vi "smartmeshIP serial mux check connection.vi"(8 "error in":errorcluster, 11 "serial mux adress":T1={"serial_mux IP"="127.0.0.1", "rserial_mux port"=9900}) -> (0 "error out":errorcluster, 3 "last error out connection":errorcluster)   [LabVIEW 2017]
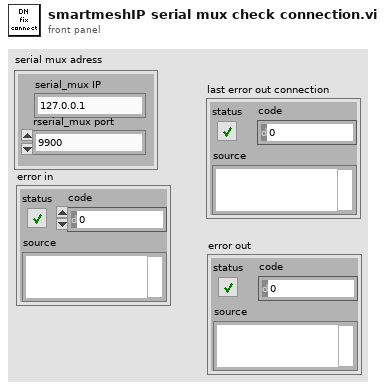
[diagram p1: front panel]
types:
  T1 = cluster{"serial_mux IP":string, "rserial_mux port":u16}
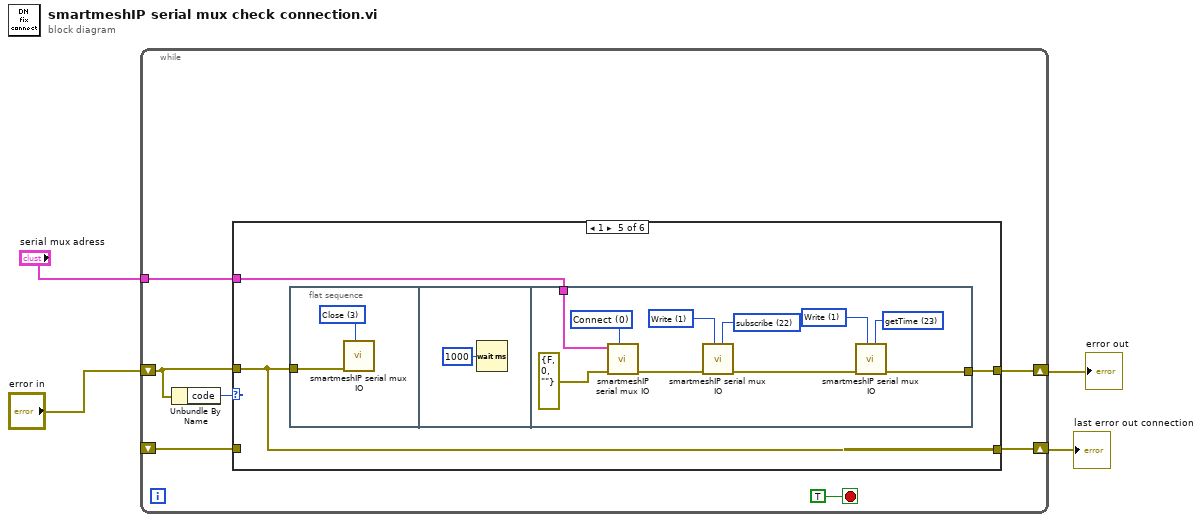
[diagram p0: block diagram]
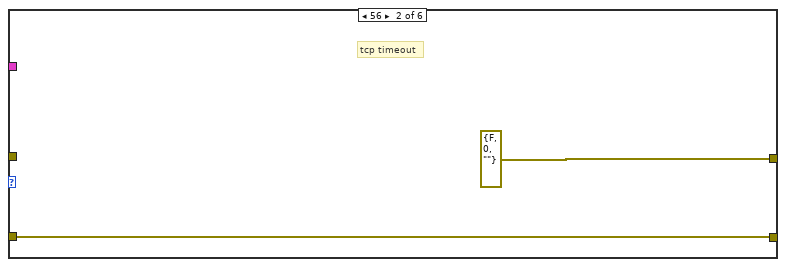
[diagram p3: hidden frame]
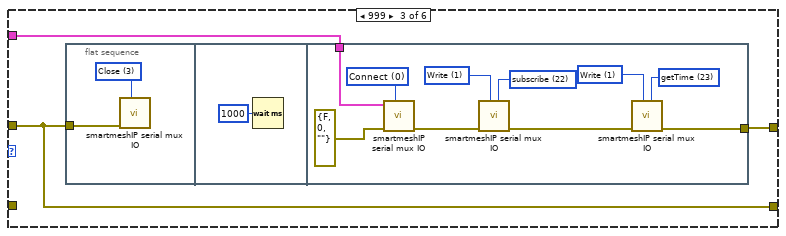
[diagram p4: hidden frame]
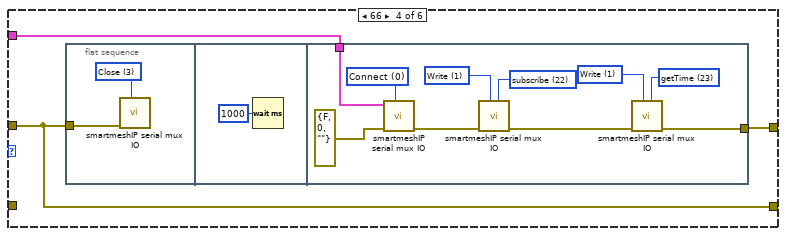
[diagram p5: hidden frame]
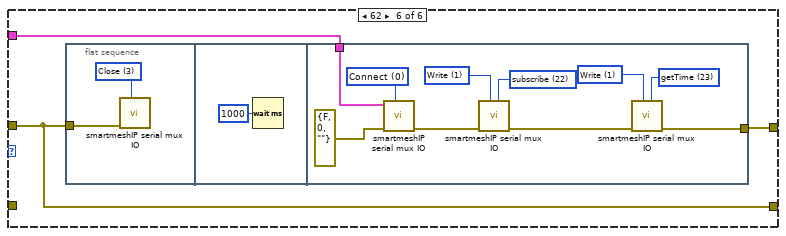
[diagram p6: hidden frame]
diagram:
  n1 = while {
    tunnel: "serial mux adress" -> [w9]
    shift-right: [w11] -> w4
    shift-left: "error in" -> [w8]
    shift-right: [w6] -> w1
    shift-left: _ -> [w5]
    stop <- TRUE stop-if-true
    n2 = Unbundle By Name(w8) -> ("code"=w10:i32)
    n3 = case shown="1" w10 {
      tunnel: [w13 errorcluster {"status"=FALSE, "code"=0, "source"=""} ("error out") w18 w34 w50 w66] -> w11
      tunnel: w8 -> [w13 _ w16 w32 w48 w64]
      tunnel: w9 -> [_ _ w17 w33 w49 w65]
      tunnel: [w12 w14 w16 w32 w48 w64] -> w6
      tunnel: w5 -> [w12 w14 _ _ _ _]
      frame 0, Default {
      }
      frame 56 {
        # "tcp timeout"
      }
      frame 999 {
        n4 = flat-sequence {
          tunnel: w16 -> [w19]
          tunnel: [w25] -> w18
          tunnel: w17 -> [w30]
          frame #0 {
            w20 = u16 3 items=["Connect", "Write", "Read", "Close"] ("State")
            n5 = call "smartmeshIP serial mux IO.vi"("State"=w20, "error in"=w19) -> ()  [unwired: 4 in, 6 out]
          }
          frame #1 {
            n6 = Wait (ms)(milliseconds to wait=u32 1000) -> ()  [unwired: 1 out]
          }
          frame #2 {
            w23 = u8 23 items=["subscribe"=22, "startNetwork"=45, "setUser"=58, "setTime"=54, "setNetworkConfig"=26, "setLicense"=56, "setIPConfig"=68, "setDownstreamFrameMode"=51, "setCommonJoinKey"=66, "setAdvertising"=50, "setACLEntry"=39, "sendIP"=59, "sendData"=44, "restorFactoryDefaults"=61, "reset"=21, "radiotestTx"=35, "radiotestRx"=37, "pingMote"=42, "getTime"=23, "getSystemInfo"=46, "radiotestStatistics"=38, "getPathInfo"=48, "getNextPath"=49, "getNextACLEntry"=40, "getNetworkInfo"=64, "getNetworkConfig"=63, "getMoteLinks"=70, "getMoteInfo"=62, "getMoteConfigByld"=65, "getMoteConfig"=47, "getManagerStatistics"=53, "getLog"=43, "getLicense"=55, "getIPConfig"=67, "exchangeNetworkID"=34, "exchangeMoteJoinKey"=33, "deleteMote"=69, "deleteACLEntry"=41, "clearStatistics"=31] ("tx_commandType")
            w24 = u16 1 items=["Connect", "Write", "Read", "Close"] ("State")
            w27 = u8 22 items=["subscribe"=22, "startNetwork"=45, "setUser"=58, "setTime"=54, "setNetworkConfig"=26, "setLicense"=56, "setIPConfig"=68, "setDownstreamFrameMode"=51, "setCommonJoinKey"=66, "setAdvertising"=50, "setACLEntry"=39, "sendIP"=59, "sendData"=44, "restorFactoryDefaults"=61, "reset"=21, "radiotestTx"=35, "radiotestRx"=37, "pingMote"=42, "getTime"=23, "getSystemInfo"=46, "radiotestStatistics"=38, "getPathInfo"=48, "getNextPath"=49, "getNextACLEntry"=40, "getNetworkInfo"=64, "getNetworkConfig"=63, "getMoteLinks"=70, "getMoteInfo"=62, "getMoteConfigByld"=65, "getMoteConfig"=47, "getManagerStatistics"=53, "getLog"=43, "getLicense"=55, "getIPConfig"=67, "exchangeNetworkID"=34, "exchangeMoteJoinKey"=33, "deleteMote"=69, "deleteACLEntry"=41, "clearStatistics"=31] ("tx_commandType")
            w28 = u16 1 items=["Connect", "Write", "Read", "Close"] ("State")
            w29 = u16 0 items=["Connect", "Write", "Read", "Close"] ("State")
            n7 = call "smartmeshIP serial mux IO.vi"("State"=w29, "error in"=errorcluster {"status"=FALSE, "code"=0, "source"=""}, "serial mux adress"=w30) -> ("error out"=w31:errorcluster)  [unwired: 3 in, 5 out]
            n8 = call "smartmeshIP serial mux IO.vi"("tx_commandType"=w27, "State"=w28, "error in"=w31) -> ("error out"=w26:errorcluster)  [unwired: 3 in, 5 out]
            n9 = call "smartmeshIP serial mux IO.vi"("tx_commandType"=w23, "State"=w24, "error in"=w26) -> ("error out"=w25:errorcluster)  [unwired: 3 in, 5 out]
          }
        }
      }
      frame 66 {
        n10 = flat-sequence {
          tunnel: w32 -> [w35]
          tunnel: [w41] -> w34
          tunnel: w33 -> [w46]
          frame #0 {
            w36 = u16 3 items=["Connect", "Write", "Read", "Close"] ("State")
            n11 = call "smartmeshIP serial mux IO.vi"("State"=w36, "error in"=w35) -> ()  [unwired: 4 in, 6 out]
          }
          frame #1 {
            n12 = Wait (ms)(milliseconds to wait=u32 1000) -> ()  [unwired: 1 out]
          }
          frame #2 {
            w39 = u8 23 items=["subscribe"=22, "startNetwork"=45, "setUser"=58, "setTime"=54, "setNetworkConfig"=26, "setLicense"=56, "setIPConfig"=68, "setDownstreamFrameMode"=51, "setCommonJoinKey"=66, "setAdvertising"=50, "setACLEntry"=39, "sendIP"=59, "sendData"=44, "restorFactoryDefaults"=61, "reset"=21, "radiotestTx"=35, "radiotestRx"=37, "pingMote"=42, "getTime"=23, "getSystemInfo"=46, "radiotestStatistics"=38, "getPathInfo"=48, "getNextPath"=49, "getNextACLEntry"=40, "getNetworkInfo"=64, "getNetworkConfig"=63, "getMoteLinks"=70, "getMoteInfo"=62, "getMoteConfigByld"=65, "getMoteConfig"=47, "getManagerStatistics"=53, "getLog"=43, "getLicense"=55, "getIPConfig"=67, "exchangeNetworkID"=34, "exchangeMoteJoinKey"=33, "deleteMote"=69, "deleteACLEntry"=41, "clearStatistics"=31] ("tx_commandType")
            w40 = u16 1 items=["Connect", "Write", "Read", "Close"] ("State")
            w43 = u8 22 items=["subscribe"=22, "startNetwork"=45, "setUser"=58, "setTime"=54, "setNetworkConfig"=26, "setLicense"=56, "setIPConfig"=68, "setDownstreamFrameMode"=51, "setCommonJoinKey"=66, "setAdvertising"=50, "setACLEntry"=39, "sendIP"=59, "sendData"=44, "restorFactoryDefaults"=61, "reset"=21, "radiotestTx"=35, "radiotestRx"=37, "pingMote"=42, "getTime"=23, "getSystemInfo"=46, "radiotestStatistics"=38, "getPathInfo"=48, "getNextPath"=49, "getNextACLEntry"=40, "getNetworkInfo"=64, "getNetworkConfig"=63, "getMoteLinks"=70, "getMoteInfo"=62, "getMoteConfigByld"=65, "getMoteConfig"=47, "getManagerStatistics"=53, "getLog"=43, "getLicense"=55, "getIPConfig"=67, "exchangeNetworkID"=34, "exchangeMoteJoinKey"=33, "deleteMote"=69, "deleteACLEntry"=41, "clearStatistics"=31] ("tx_commandType")
            w44 = u16 1 items=["Connect", "Write", "Read", "Close"] ("State")
            w45 = u16 0 items=["Connect", "Write", "Read", "Close"] ("State")
            n13 = call "smartmeshIP serial mux IO.vi"("State"=w45, "error in"=errorcluster {"status"=FALSE, "code"=0, "source"=""}, "serial mux adress"=w46) -> ("error out"=w47:errorcluster)  [unwired: 3 in, 5 out]
            n14 = call "smartmeshIP serial mux IO.vi"("tx_commandType"=w43, "State"=w44, "error in"=w47) -> ("error out"=w42:errorcluster)  [unwired: 3 in, 5 out]
            n15 = call "smartmeshIP serial mux IO.vi"("tx_commandType"=w39, "State"=w40, "error in"=w42) -> ("error out"=w41:errorcluster)  [unwired: 3 in, 5 out]
          }
        }
      }
      frame 1 {
        n16 = flat-sequence {
          tunnel: w48 -> [w51]
          tunnel: [w57] -> w50
          tunnel: w49 -> [w62]
          frame #0 {
            w52 = u16 3 items=["Connect", "Write", "Read", "Close"] ("State")
            n17 = call "smartmeshIP serial mux IO.vi"("State"=w52, "error in"=w51) -> ()  [unwired: 4 in, 6 out]
          }
          frame #1 {
            n18 = Wait (ms)(milliseconds to wait=u32 1000) -> ()  [unwired: 1 out]
          }
          frame #2 {
            w55 = u8 23 items=["subscribe"=22, "startNetwork"=45, "setUser"=58, "setTime"=54, "setNetworkConfig"=26, "setLicense"=56, "setIPConfig"=68, "setDownstreamFrameMode"=51, "setCommonJoinKey"=66, "setAdvertising"=50, "setACLEntry"=39, "sendIP"=59, "sendData"=44, "restorFactoryDefaults"=61, "reset"=21, "radiotestTx"=35, "radiotestRx"=37, "pingMote"=42, "getTime"=23, "getSystemInfo"=46, "radiotestStatistics"=38, "getPathInfo"=48, "getNextPath"=49, "getNextACLEntry"=40, "getNetworkInfo"=64, "getNetworkConfig"=63, "getMoteLinks"=70, "getMoteInfo"=62, "getMoteConfigByld"=65, "getMoteConfig"=47, "getManagerStatistics"=53, "getLog"=43, "getLicense"=55, "getIPConfig"=67, "exchangeNetworkID"=34, "exchangeMoteJoinKey"=33, "deleteMote"=69, "deleteACLEntry"=41, "clearStatistics"=31] ("tx_commandType")
            w56 = u16 1 items=["Connect", "Write", "Read", "Close"] ("State")
            w59 = u8 22 items=["subscribe"=22, "startNetwork"=45, "setUser"=58, "setTime"=54, "setNetworkConfig"=26, "setLicense"=56, "setIPConfig"=68, "setDownstreamFrameMode"=51, "setCommonJoinKey"=66, "setAdvertising"=50, "setACLEntry"=39, "sendIP"=59, "sendData"=44, "restorFactoryDefaults"=61, "reset"=21, "radiotestTx"=35, "radiotestRx"=37, "pingMote"=42, "getTime"=23, "getSystemInfo"=46, "radiotestStatistics"=38, "getPathInfo"=48, "getNextPath"=49, "getNextACLEntry"=40, "getNetworkInfo"=64, "getNetworkConfig"=63, "getMoteLinks"=70, "getMoteInfo"=62, "getMoteConfigByld"=65, "getMoteConfig"=47, "getManagerStatistics"=53, "getLog"=43, "getLicense"=55, "getIPConfig"=67, "exchangeNetworkID"=34, "exchangeMoteJoinKey"=33, "deleteMote"=69, "deleteACLEntry"=41, "clearStatistics"=31] ("tx_commandType")
            w60 = u16 1 items=["Connect", "Write", "Read", "Close"] ("State")
            w61 = u16 0 items=["Connect", "Write", "Read", "Close"] ("State")
            n19 = call "smartmeshIP serial mux IO.vi"("State"=w61, "error in"=errorcluster {"status"=FALSE, "code"=0, "source"=""}, "serial mux adress"=w62) -> ("error out"=w63:errorcluster)  [unwired: 3 in, 5 out]
            n20 = call "smartmeshIP serial mux IO.vi"("tx_commandType"=w59, "State"=w60, "error in"=w63) -> ("error out"=w58:errorcluster)  [unwired: 3 in, 5 out]
            n21 = call "smartmeshIP serial mux IO.vi"("tx_commandType"=w55, "State"=w56, "error in"=w58) -> ("error out"=w57:errorcluster)  [unwired: 3 in, 5 out]
          }
        }
      }
      frame 62 {
        n22 = flat-sequence {
          tunnel: w64 -> [w67]
          tunnel: [w73] -> w66
          tunnel: w65 -> [w78]
          frame #0 {
            w68 = u16 3 items=["Connect", "Write", "Read", "Close"] ("State")
            n23 = call "smartmeshIP serial mux IO.vi"("State"=w68, "error in"=w67) -> ()  [unwired: 4 in, 6 out]
          }
          frame #1 {
            n24 = Wait (ms)(milliseconds to wait=u32 1000) -> ()  [unwired: 1 out]
          }
          frame #2 {
            w71 = u8 23 items=["subscribe"=22, "startNetwork"=45, "setUser"=58, "setTime"=54, "setNetworkConfig"=26, "setLicense"=56, "setIPConfig"=68, "setDownstreamFrameMode"=51, "setCommonJoinKey"=66, "setAdvertising"=50, "setACLEntry"=39, "sendIP"=59, "sendData"=44, "restorFactoryDefaults"=61, "reset"=21, "radiotestTx"=35, "radiotestRx"=37, "pingMote"=42, "getTime"=23, "getSystemInfo"=46, "radiotestStatistics"=38, "getPathInfo"=48, "getNextPath"=49, "getNextACLEntry"=40, "getNetworkInfo"=64, "getNetworkConfig"=63, "getMoteLinks"=70, "getMoteInfo"=62, "getMoteConfigByld"=65, "getMoteConfig"=47, "getManagerStatistics"=53, "getLog"=43, "getLicense"=55, "getIPConfig"=67, "exchangeNetworkID"=34, "exchangeMoteJoinKey"=33, "deleteMote"=69, "deleteACLEntry"=41, "clearStatistics"=31] ("tx_commandType")
            w72 = u16 1 items=["Connect", "Write", "Read", "Close"] ("State")
            w75 = u8 22 items=["subscribe"=22, "startNetwork"=45, "setUser"=58, "setTime"=54, "setNetworkConfig"=26, "setLicense"=56, "setIPConfig"=68, "setDownstreamFrameMode"=51, "setCommonJoinKey"=66, "setAdvertising"=50, "setACLEntry"=39, "sendIP"=59, "sendData"=44, "restorFactoryDefaults"=61, "reset"=21, "radiotestTx"=35, "radiotestRx"=37, "pingMote"=42, "getTime"=23, "getSystemInfo"=46, "radiotestStatistics"=38, "getPathInfo"=48, "getNextPath"=49, "getNextACLEntry"=40, "getNetworkInfo"=64, "getNetworkConfig"=63, "getMoteLinks"=70, "getMoteInfo"=62, "getMoteConfigByld"=65, "getMoteConfig"=47, "getManagerStatistics"=53, "getLog"=43, "getLicense"=55, "getIPConfig"=67, "exchangeNetworkID"=34, "exchangeMoteJoinKey"=33, "deleteMote"=69, "deleteACLEntry"=41, "clearStatistics"=31] ("tx_commandType")
            w76 = u16 1 items=["Connect", "Write", "Read", "Close"] ("State")
            w77 = u16 0 items=["Connect", "Write", "Read", "Close"] ("State")
            n25 = call "smartmeshIP serial mux IO.vi"("State"=w77, "error in"=errorcluster {"status"=FALSE, "code"=0, "source"=""}, "serial mux adress"=w78) -> ("error out"=w79:errorcluster)  [unwired: 3 in, 5 out]
            n26 = call "smartmeshIP serial mux IO.vi"("tx_commandType"=w75, "State"=w76, "error in"=w79) -> ("error out"=w74:errorcluster)  [unwired: 3 in, 5 out]
            n27 = call "smartmeshIP serial mux IO.vi"("tx_commandType"=w71, "State"=w72, "error in"=w74) -> ("error out"=w73:errorcluster)  [unwired: 3 in, 5 out]
          }
        }
      }
    }
  }
  "error out" <- w4
  "last error out connection" <- w1
